vi "Get Error.vi"(9 "Actual Angle":dbl format="%#_13g", 10 "Desired Angle":dbl format="%#_13g", 11 "Motor Power":dbl format="%#_13g") -> (2 "Motor Power":dbl format="%#_13g", 3 "Angle Error":dbl format="%#_13g")   [LabVIEW 2018]
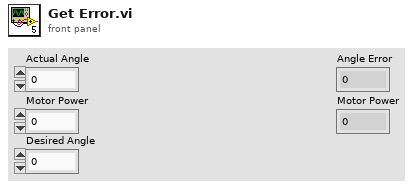
[diagram p1: front panel]
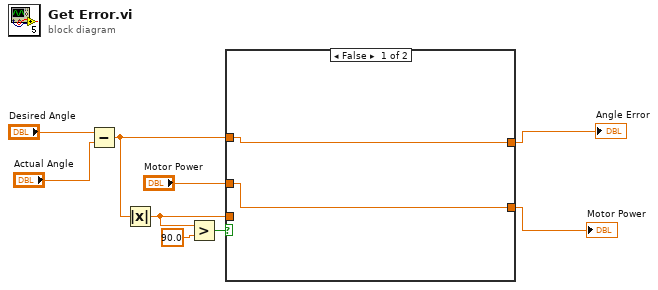
[diagram p0: block diagram]
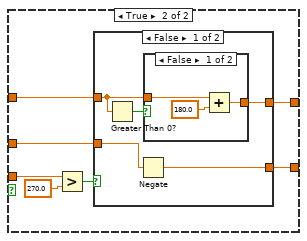
[diagram p2: hidden frame]
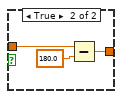
[diagram p3: hidden frame]
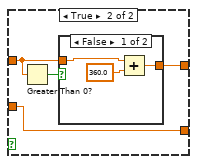
[diagram p4: hidden frame]
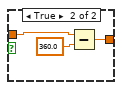
[diagram p5: hidden frame]
diagram:
  n1 = Subtract(x="Desired Angle", y="Actual Angle") -> (x-y=w3:dbl)
  n2 = Absolute Value(x=w3) -> (abs(x)=w6:dbl)
  n3 = Greater?(x=w6, y=90.0) -> (0:w4:bool)
  n4 = case shown="False" w4 {
    tunnel: "Motor Power" -> [w10 w14]
    tunnel: w6 -> [_ w18]
    tunnel: w3 -> [w11 w15]
    tunnel: [w11 w13] -> w2
    tunnel: [w10 w12] -> w1
    frame False {
    }
    frame True {
      n5 = Greater?(x=w18, y=270.0) -> (0:w16:bool)
      n6 = case shown="False" w16 {
        tunnel: w15 -> [w20 w32]
        tunnel: w14 -> [w22 w30]
        tunnel: [w19 w31] -> w13
        tunnel: [w21 w30] -> w12
        frame False {
          n7 = Greater Than 0?(x=w20) -> (x > 0?=w23:bool)
          n8 = Negate(x=w22) -> (-x=w21:dbl)
          n9 = case shown="False" w23 {
            tunnel: w20 -> [w26 w29]
            tunnel: [w24 w27] -> w19
            frame False {
              n10 = Add(x=w26, y=180.0) -> (x+y=w24:dbl)
            }
            frame True {
              n11 = Subtract(x=w29, y=180.0) -> (x-y=w27:dbl)
            }
          }
        }
        frame True {
          n12 = Greater Than 0?(x=w32) -> (x > 0?=w33:bool)
          n13 = case shown="False" w33 {
            tunnel: w32 -> [w36 w39]
            tunnel: [w34 w37] -> w31
            frame False {
              n14 = Add(x=w36, y=360.0) -> (x+y=w34:dbl)
            }
            frame True {
              n15 = Subtract(x=w39, y=360.0) -> (x-y=w37:dbl)
            }
          }
        }
      }
    }
  }
  "Angle Error" <- w2
  "Motor Power" <- w1
